vi "UpdateTestStatus.vi"(0 "GUI_Handler_Seq in":refnum<class "GUI_Handler_Seq.lvclass">, 5 "TestMeasureStep in":refnum<class "TestMeasureStep.lvclass">, 11 "error in (no error)":errorcluster) -> (4 "GUI_Handler_Seq out":refnum<class "GUI_Handler_Seq.lvclass">, 15 "error out":errorcluster)   [LabVIEW 2017, in "GUI_Handler_Seq.lvclass"]
uses:
  GUI_Handler_Seq.lvclass
  TestMeasureStep/TestMeasureStep.lvclass
  TestMeasureStep/TestMeasureStep.lvclass/TestMeasureStep.ctl
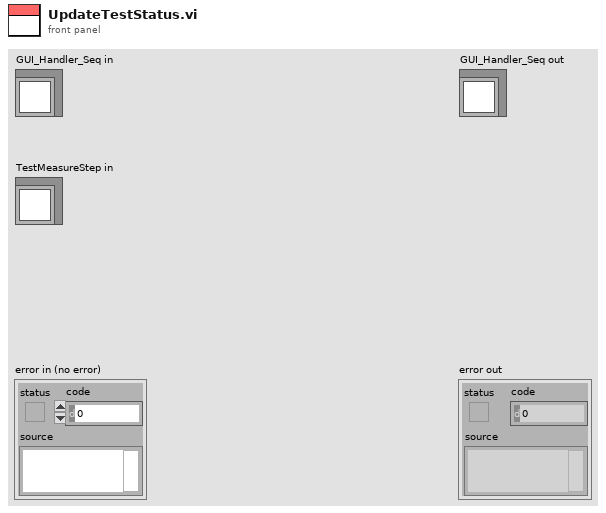
[diagram p1: front panel]
types:
  T1 = typedef "TestSeqClass.lvclass/TesstepType.ctl" = cluster{"TestName":string, "Meas":dbl, "Min ":dbl, "Max":dbl, "TestStatus":T2, "StringLimit":string, "StringMeas":string, "Unit":string}
  T2 = typedef "TestStatus.ctl" = enum16{"Not Executed", "Passed", "Failed", "Inconclusive", "Processing"}
  T3 = cluster{"IndexInList":u32, "new element/subarray":i32}
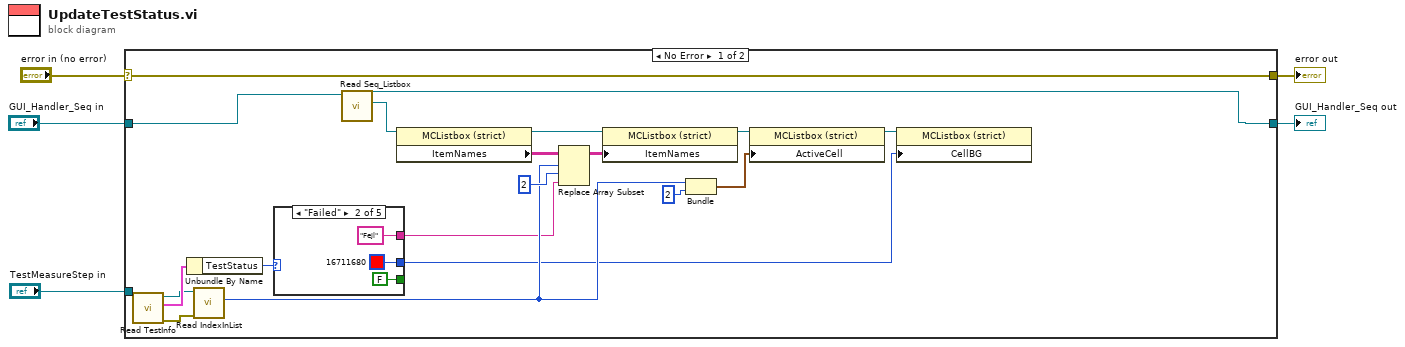
[diagram p0: block diagram]
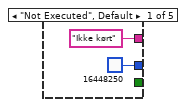
[diagram p2: hidden frame]
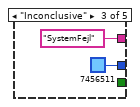
[diagram p3: hidden frame]
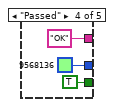
[diagram p4: hidden frame]
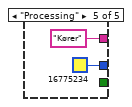
[diagram p5: hidden frame]
diagram:
  n1 = case shown="No Error" "error in (no error)" {
    selector: "error in (no error)" -> [w25 w39]
    tunnel: [w25 w39] -> w4
    tunnel: [w6 w38] -> w2
    tunnel: "GUI_Handler_Seq in" -> [w24 w38]
    tunnel: "TestMeasureStep in" -> [w10 _]
    frame No Error {
      n2 = call-dynamic "Read TestInfo.vi"("TestMeasureStep in"=w10) -> ("error out"=w13:errorcluster, "TestInfo 2"=w15:T1, "TestMeasureStep out"=w12:refnum<class "TestMeasureStep.lvclass">)  [unwired: 8 in]
      n3 = Unbundle By Name(w15) -> ("TestStatus"=w14:T2)
      n4 = call "Read IndexInList.vi"("error in (no error)"=w13, "TestMeasureStep in"=w12) -> ("IndexInList"=w11:u32)  [unwired: 7 in, 2 out]
      n5 = case shown="\"Failed\"" w14 {
        tunnel: [u32 16448250 ("Active Cell:Cell Background Color") u32 16711680 ("Active Cell:Cell Background Color") u32 7456511 ("Active Cell:Cell Background Color") u32 9568136 ("Active Cell:Cell Background Color") u32 16775234 ("Active Cell:Cell Background Color")] -> w9
        tunnel: ["Ikke kørt" ("new element/subarray") "Fejl" ("new element/subarray") "SystemFejl" ("new element/subarray") "OK" ("new element/subarray") "Kører" ("new element/subarray")] -> w7
        tunnel: [_ FALSE _ TRUE _] -> _
        frame "Not Executed", Default {
        }
        frame "Failed" {
        }
        frame "Inconclusive" {
        }
        frame "Passed" {
        }
        frame "Processing" {
        }
      }
      n6 = call-dynamic "Read Seq_Listbox.vi"("GUI_Handler_Seq in"=w24) -> ("Seq_Listbox"=w23:refnum<vi>, "GUI_Handler_Seq out"=w6:refnum<class "GUI_Handler_Seq.lvclass">)  [unwired: 8 in, 1 out]
      n7 = property class="MCListbox (strict)"(reference=w23) -> (reference out=w21:refnum<vi>, "ItemNames"=w22:string[][])  [unwired: 1 in, 1 out]
      n8 = Replace Array Subset(array=w22, new element=w7, index (row)=w11, index (col)=2 ("disabled index (col)")) -> (w20:string[][])
      n9 = property class="MCListbox (strict)"(reference=w21, "ItemNames"=w20) -> (reference out=w19:refnum<vi>)  [unwired: 1 in, 1 out]
      n10 = Bundle("IndexInList"=w11, "new element/subarray"=2) -> (w16:T3)  [unwired: 1 in]
      n11 = property class="MCListbox (strict)"(reference=w19, "ActiveCell"=w16) -> (reference out=w8:refnum<vi>)  [unwired: 1 in, 1 out]
      n12 = property class="MCListbox (strict)"(reference=w8, "CellBG"=w9) -> ()  [unwired: 1 in, 2 out]
    }
    frame Error {
    }
  }
  "error out" <- w4
  "GUI_Handler_Seq out" <- w2
